vi "SCPE.vi"() -> ()   [LabVIEW 2020]
uses:
  <vilib>/Utility/file.llb/Read Delimited Spreadsheet (DBL).vi
panel:
  out "Rs":dbl
  out "Rsh":dbl
  out "Voc":dbl
  out "Isc":dbl
  in  "file path (dialog if empty)":path
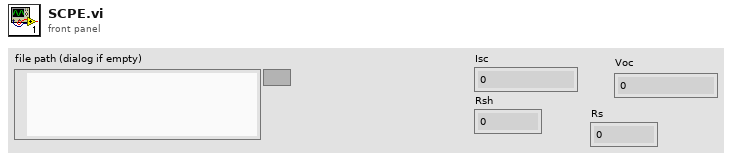
[diagram p1: front panel]
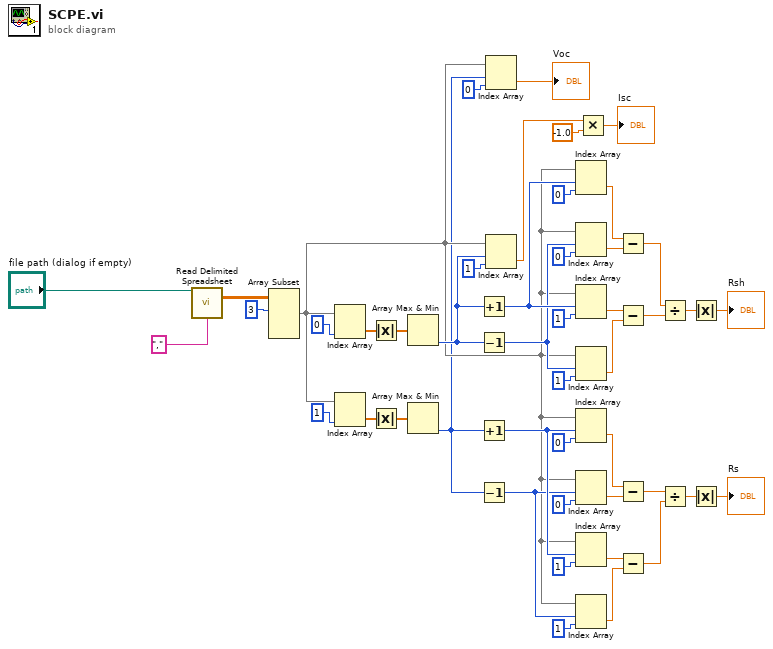
[diagram p0: block diagram]
diagram:
  n1 = call-poly <vilib>:"Read Delimited Spreadsheet.vi"("file path (dialog if empty)"="file path (dialog if empty)", "delimiter (\\t)"="," ("delimiter (\\t)")) -> ("all rows"=w45:dbl[][])  [unwired: 8 in, 5 out]
  n2 = Array Subset(array=w45, index (row)=3 ("index")) -> (w2:dbl[][])  [unwired: 3 in]
  n3 = Index Array(array=w2, index (col)=0 ("disabled index (col)")) -> (element=w42:dbl[])  [unwired: 1 in]
  n4 = Index Array(array=w2, index (col)=1 ("disabled index (col)")) -> (element=w35:dbl[])  [unwired: 1 in]
  n5 = Absolute Value(x=w42) -> (abs(x)=w41:dbl[])
  n6 = Absolute Value(x=w35) -> (abs(x)=w34:dbl[])
  n7 = Array Max & Min(array=w41) -> (min index (indices)=w31:i32)  [unwired: 3 out]
  n8 = Array Max & Min(array=w34) -> (min index (indices)=w1:i32)  [unwired: 3 out]
  n9 = Increment(x=w31) -> (x+1=w30:i32)
  n10 = Decrement(x=w31) -> (x-1=w25:i32)
  n11 = Increment(x=w1) -> (x+1=w16:i32)
  n12 = Decrement(x=w1) -> (x-1=w11:i32)
  n13 = Index Array(array=w2, index (row)=w1, index (col)=0 ("disabled index (col)")) -> (element=→"Voc":dbl)
  n14 = Index Array(array=w2, index (row)=w31, index (col)=1 ("disabled index (col)")) -> (element=w39:dbl)
  n15 = Index Array(array=w2, index (row)=w30, index (col)=0 ("disabled index (col)")) -> (element=w24:dbl)
  n16 = Index Array(array=w2, index (row)=w25, index (col)=0 ("disabled index (col)")) -> (element=w23:dbl)
  n17 = Index Array(array=w2, index (row)=w30, index (col)=1 ("disabled index (col)")) -> (element=w22:dbl)
  n18 = Index Array(array=w2, index (row)=w25, index (col)=1 ("disabled index (col)")) -> (element=w21:dbl)
  n19 = Index Array(array=w2, index (row)=w16, index (col)=0 ("disabled index (col)")) -> (element=w10:dbl)
  n20 = Index Array(array=w2, index (row)=w11, index (col)=0 ("disabled index (col)")) -> (element=w9:dbl)
  n21 = Index Array(array=w2, index (row)=w16, index (col)=1 ("disabled index (col)")) -> (element=w8:dbl)
  n22 = Index Array(array=w2, index (row)=w11, index (col)=1 ("disabled index (col)")) -> (element=w7:dbl)
  n23 = Multiply(x=w39, y=-1.0) -> (x*y=→"Isc":dbl)
  n24 = Subtract(x=w24, y=w23) -> (x-y=w20:dbl)
  n25 = Subtract(x=w22, y=w21) -> (x-y=w19:dbl)
  n26 = Subtract(x=w10, y=w9) -> (x-y=w6:dbl)
  n27 = Subtract(x=w8, y=w7) -> (x-y=w5:dbl)
  n28 = Divide(x=w20, y=w19) -> (x/y=w18:dbl)
  n29 = Divide(x=w6, y=w5) -> (x/y=w4:dbl)
  n30 = Absolute Value(x=w18) -> (abs(x)=→"Rsh":dbl)
  n31 = Absolute Value(x=w4) -> (abs(x)=→"Rs":dbl)
